vi "Actor Core.vi"(8 "error in":errorcluster, 11 "Side Menu in":refnum<class "Side Menu.lvclass">) -> (0 "error out":errorcluster, 3 "Actor out":refnum<class "Actor.lvclass">)   [LabVIEW 2020, in "Side Menu View.lvlib" / "Side Menu.lvclass"]
doc: "(<B>Filename</B>: Actor Framework.lvlib:Actor.lvclass:Actor Core.vi)\n\nReceives messages to the actor, reacts to them, and initiates any error handling that may shut the actor down.\n\nDescendant classes may override this VI to append parallel tasks for the actor to complete while it handles messages. Overrides use the Call Parent Method node."
uses:
  Side Menu.lvclass
  C:/Program Files/National Instruments/LabVIEW 2020/vi.lib/ActorFramework/Actor/Actor.lvclass
  <vilib>/ActorFramework/Actor/Actor.lvclass
  <vilib>/ActorFramework/Actor/Actor.lvclass/Actor.ctl
  <vilib>/Utility/miscctls.llb/LVPositionTypeDef.ctl
  <vilib>/ActorFrameworkMVC/View Controller/View Controller Messages/Move Subpanel Msg/Move Subpanel Msg.lvclass/Move Subpanel Msg.ctl
  <vilib>/ActorFramework/Message Enqueuer/Message Enqueuer.lvclass/Message Enqueuer.ctl
  <vilib>/ActorFrameworkMVC/View Controller/View Controller Messages/Insert Subpanel Msg/Insert Subpanel Msg.lvclass/Insert Subpanel Msg.ctl
  <vilib>/ActorFramework/Message Enqueuer/Enqueue.vi
  <vilib>/ActorFrameworkMVC/View Controller/View Controller Messages/Move Subpanel Msg/Move Subpanel Msg.lvclass
  C:/Program Files/National Instruments/LabVIEW 2020/vi.lib/ActorFramework/Message/Message.lvclass
  <vilib>/ActorFrameworkMVC/View Controller/View Controller Messages/Insert Subpanel Msg/Insert Subpanel Msg.lvclass
  UI Controller/UI Controller Messages/Initialize Subpanels Msg/Initialize Subpanels Msg.lvclass
  <vilib>/ActorFramework/Message Priority Queue/Priority Enqueue.vi
  <vilib>/ActorFrameworkMVC/Abstract View/Abstract View/Abstract View.lvclass
panel:
  in  "Print Menu Button":bool
  in  "Save As Menu Button":bool
  in  "Save Menu Button":bool
  in  "Create Document Menu Button":bool
  in  "Menu Button":bool=TRUE
  in  "Settings Menu Button":bool
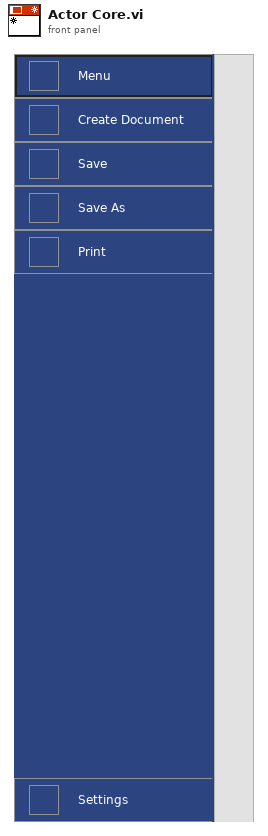
[diagram p1: front panel]
types:
  T1 = typedef "LVPositionTypeDef.ctl" = cluster{"Left":i32, "Top":i32}
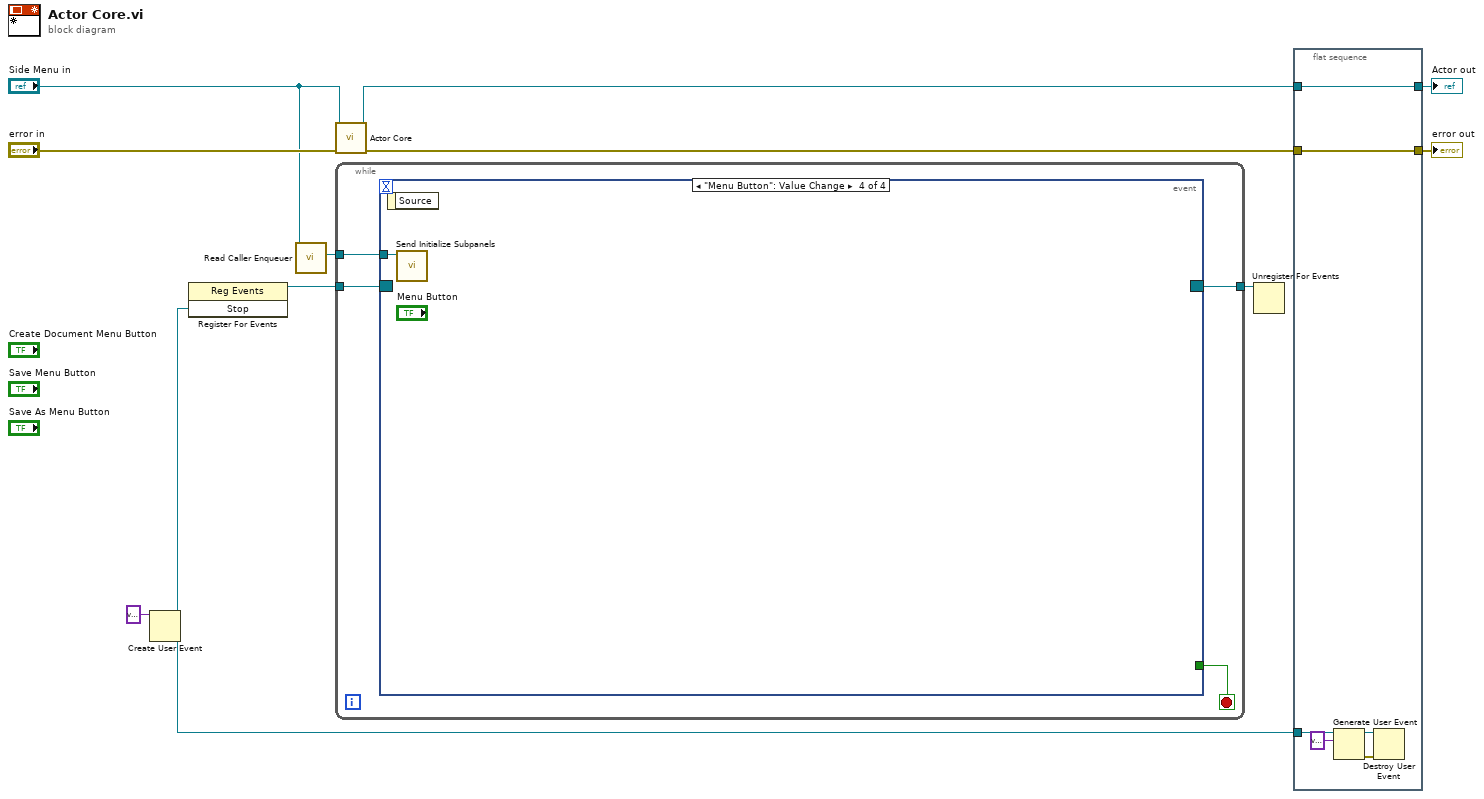
[diagram p0: block diagram]
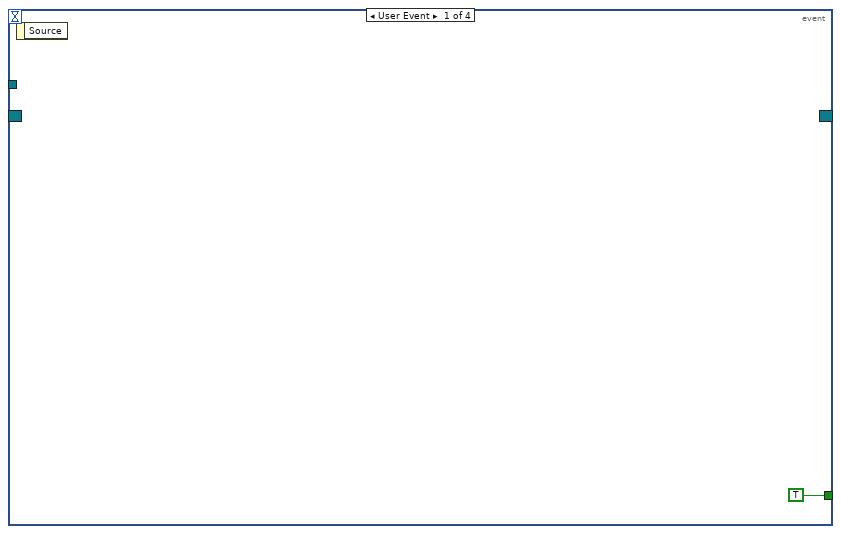
[diagram p2: hidden frame]
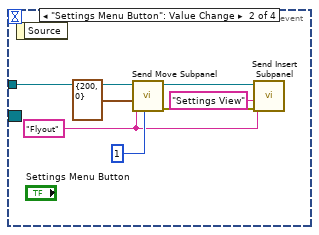
[diagram p3: hidden frame]
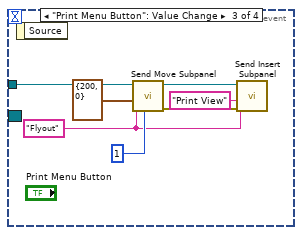
[diagram p4: hidden frame]
diagram:
  n1 = Create User Event(user event datatype=variant ("Stop")) -> (user event=w5:refnum<user-event>)  [unwired: 1 in, 1 out]
  n2 = register-events(w5) -> (reference out=w7:refnum<event-registration>)  [unwired: 2 in, 1 out]
  n3 = call <vilib>:"Read Caller Enqueuer.vi"("Actor"="Side Menu in") -> ("Caller Enqueuer"=w9:refnum<class "Message Enqueuer.lvclass">)  [unwired: 10 in]
  n4 = call-parent "Actor Core.vi"("error in"="error in", "Abstract View in"="Side Menu in") -> ("error out"=w3:errorcluster, "Actor out"=w2:refnum<class "Actor.lvclass">)  [unwired: 8 in]
  n5 = while {
    tunnel: w9 -> [w15]
    tunnel: w7 -> [w14]
    tunnel: [w13] -> w6
    stop <- w12 stop-if-true
    n6 = event shown="[3] \"Menu Button\": Value Change" {
      selector: w14 -> [_ _ _ _]
      dyn-events: [_ _ _ _] -> w13
      timeout: _ -> [_ _ _ _]
      tunnel: w15 -> [_ w20 w27 w31]
      tunnel: [TRUE _ _ _] -> w12
      event User Event {
        n7 = event-data() -> ()  [unwired: 1 in, 1 out]
      }
      event "Settings Menu Button": Value Change {
        w17 = "Flyout" ("Subpanel Name")
        n8 = event-data() -> ()  [unwired: 1 in, 1 out]
        n9 = call <vilib>:"Send Move Subpanel.vi"("Loop Number (16)"=1, "Position"=T1 {"Left"=200, "Top"=0}, "Subpanel Name"=w17, "Message Enqueuer"=w20) -> ("error out"=w18:errorcluster, "Message Enqueuer out"=w19:refnum<class "Message Enqueuer.lvclass">)  [unwired: 6 in]
        n10 = call <vilib>:"Send Insert Subpanel.vi"("error in (no error)"=w18, "View Name"="Settings View", "Subpanel Name"=w17, "Message Enqueuer"=w19) -> ()  [unwired: 6 in, 2 out]
      }
      event "Print Menu Button": Value Change {
        w24 = "Flyout" ("Subpanel Name")
        n11 = event-data() -> ()  [unwired: 1 in, 1 out]
        n12 = call <vilib>:"Send Move Subpanel.vi"("Loop Number (16)"=1, "Position"=T1 {"Left"=200, "Top"=0}, "Subpanel Name"=w24, "Message Enqueuer"=w27) -> ("error out"=w25:errorcluster, "Message Enqueuer out"=w26:refnum<class "Message Enqueuer.lvclass">)  [unwired: 6 in]
        n13 = call <vilib>:"Send Insert Subpanel.vi"("error in (no error)"=w25, "View Name"="Print View", "Subpanel Name"=w24, "Message Enqueuer"=w26) -> ()  [unwired: 6 in, 2 out]
      }
      event "Menu Button": Value Change {
        n14 = event-data() -> ()  [unwired: 1 in, 1 out]
        n15 = call "Send Initialize Subpanels.vi"("Message Enqueuer"=w31) -> ()  [unwired: 9 in, 2 out]
      }
    }
  }
  n16 = Unregister For Events(event registration refnum=w6) -> ()  [unwired: 1 in, 1 out]
  n17 = flat-sequence {
    tunnel: w5 -> [w35]
    tunnel: [w33] -> w4
    tunnel: w3 -> [w33]
    tunnel: w2 -> [w32]
    tunnel: [w32] -> w1
    frame #0 {
      n18 = Generate User Event(user event=w35, event data cluster=variant ("event data")) -> (user event out=w37:refnum<user-event>, error out=w36:errorcluster)  [unwired: 2 in]
      n19 = Destroy User Event(user event=w37, error in=w36) -> ()  [unwired: 1 out]
    }
  }
  "error out" <- w4
  "Actor out" <- w1
